vi "main_gui.vi"(8 "error in (no error)":errorcluster) -> (0 "error out":errorcluster)   [LabVIEW 2020]
uses:
  #typedefs/#typedef_cluster_GUI_QueueData.ctl
  #typedefs/#typedef_enum_GUI_States.ctl
  #typedefs/#typedef_enum_QueueActions.ctl
  #typedefs/#typedef_enum_EventActions.ctl
  <vilib>/Utility/miscctls.llb/LVBrowseOptionsTypeDef.ctl
  #typedefs/#typedef_cluster_GUI_Data.ctl
  <vilib>/vision/Image Controls.llb/IMAQ Image.ctl
  #typedefs/#typedef_cluster_CTRL_QueueData.ctl
  #typedefs/#typedef_enum_CTRL_States.ctl
panel:
  out "File Type":string
  in  "GenConsumerError":bool
  in  "GenProducerError":bool
  in  "Analyze Button":bool
  out "ImageName":string
  in  "Next Button":bool
  in  "Previous Button":bool
  out "ImagePreview":T1(plugin-control)
  in  "Add Button":bool
  in  "Select folder or image":path
  in  "Exit Button":bool
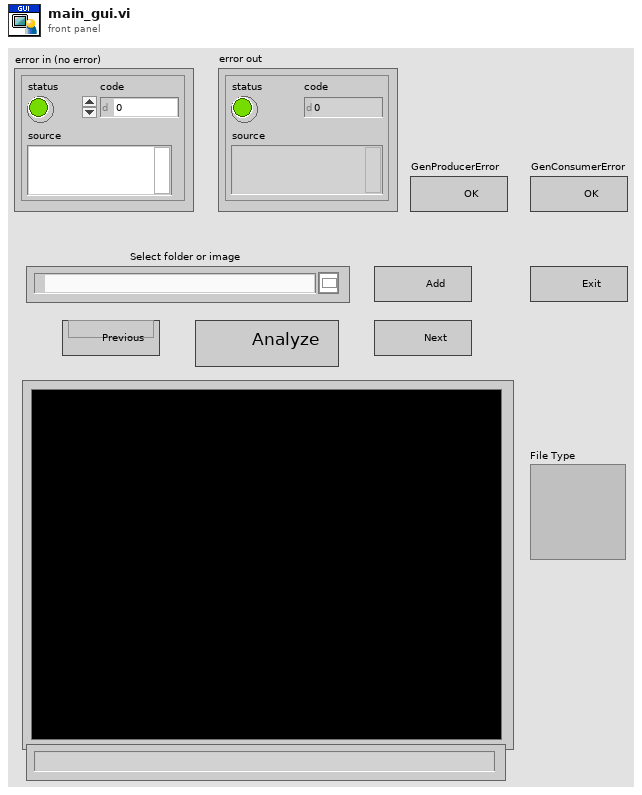
[diagram p1: front panel]
types:
  T1 = typedef "IMAQ Image.ctl" = refnum<image>
  T2 = typedef "#typedef_enum_EventActions.ctl" = enum16{"Obtain", "GetRef", "Generate", "Destroy"}
  T3 = typedef "#typedef_enum_QueueActions.ctl" = enum16{"Obtain", "GetRef", "Enqueue", "Release"}
  T4 = typedef "#typedef_cluster_GUI_QueueData.ctl" = cluster{"Cmd":T5, "Variant":variant}
  T5 = typedef "#typedef_enum_GUI_States.ctl" = enum16{"Init", "AddImages", "PreviousImage", "NextImage", "AnalyzeImage", "SaveImage", "GenFakeError", "ErrorHandling", "ExitRequest", "Exit"}
  T6 = enum32{"existing file", "new file", "new or existing file", "existing dir", "new dir", "new or existing dir", "existing file (use LLBs)", "new file (use LLBs)", "new or existing file (use LLBs)", "new or existing file or directory (use LLBs)", "existing dir (use LLBs)", "new dir (use LLBs)", "new or existing dir (use LLBs)", "existing file or dir", "new file or dir", "new or existing file or dir", "existing file or dir (use LLBs)", "new file or dir (use LLBs)"}
  T7 = typedef "LVBrowseOptionsTypeDef.ctl" = cluster{"Prompt":string, "Match Pattern":string, "Mode":enum32{"existing file", "new file", "new or existing file", "existing dir", "new dir", "new or existing dir", "existing file (use LLBs)", "new file (use LLBs)", "new or existing file (use LLBs)", "new or existing file or directory (use LLBs)", "existing dir (use LLBs)", "new dir (use LLBs)", "new or existing dir (use LLBs)", "existing file or dir", "new file or dir", "new or existing file or dir", "existing file or dir (use LLBs)", "new file or dir (use LLBs)"}, "Start Path":path, "Pattern Label":string, "Button Text":string}
  T8 = typedef "#typedef_enum_CTRL_States.ctl" = enum16{"Init", "AnalyzeImage", "SaveImage", "ErrorHandling", "ExitRequest", "Exit"}
  T9 = typedef "#typedef_cluster_CTRL_QueueData.ctl" = cluster{"Cmd":T8, "Variant":variant}
  T10 = typedef "#typedef_cluster_GUI_Data.ctl" = cluster{"Images":T1[], "PreviewIndex":i32, "AnalyzeIndex":i32, "Paths":path[]}
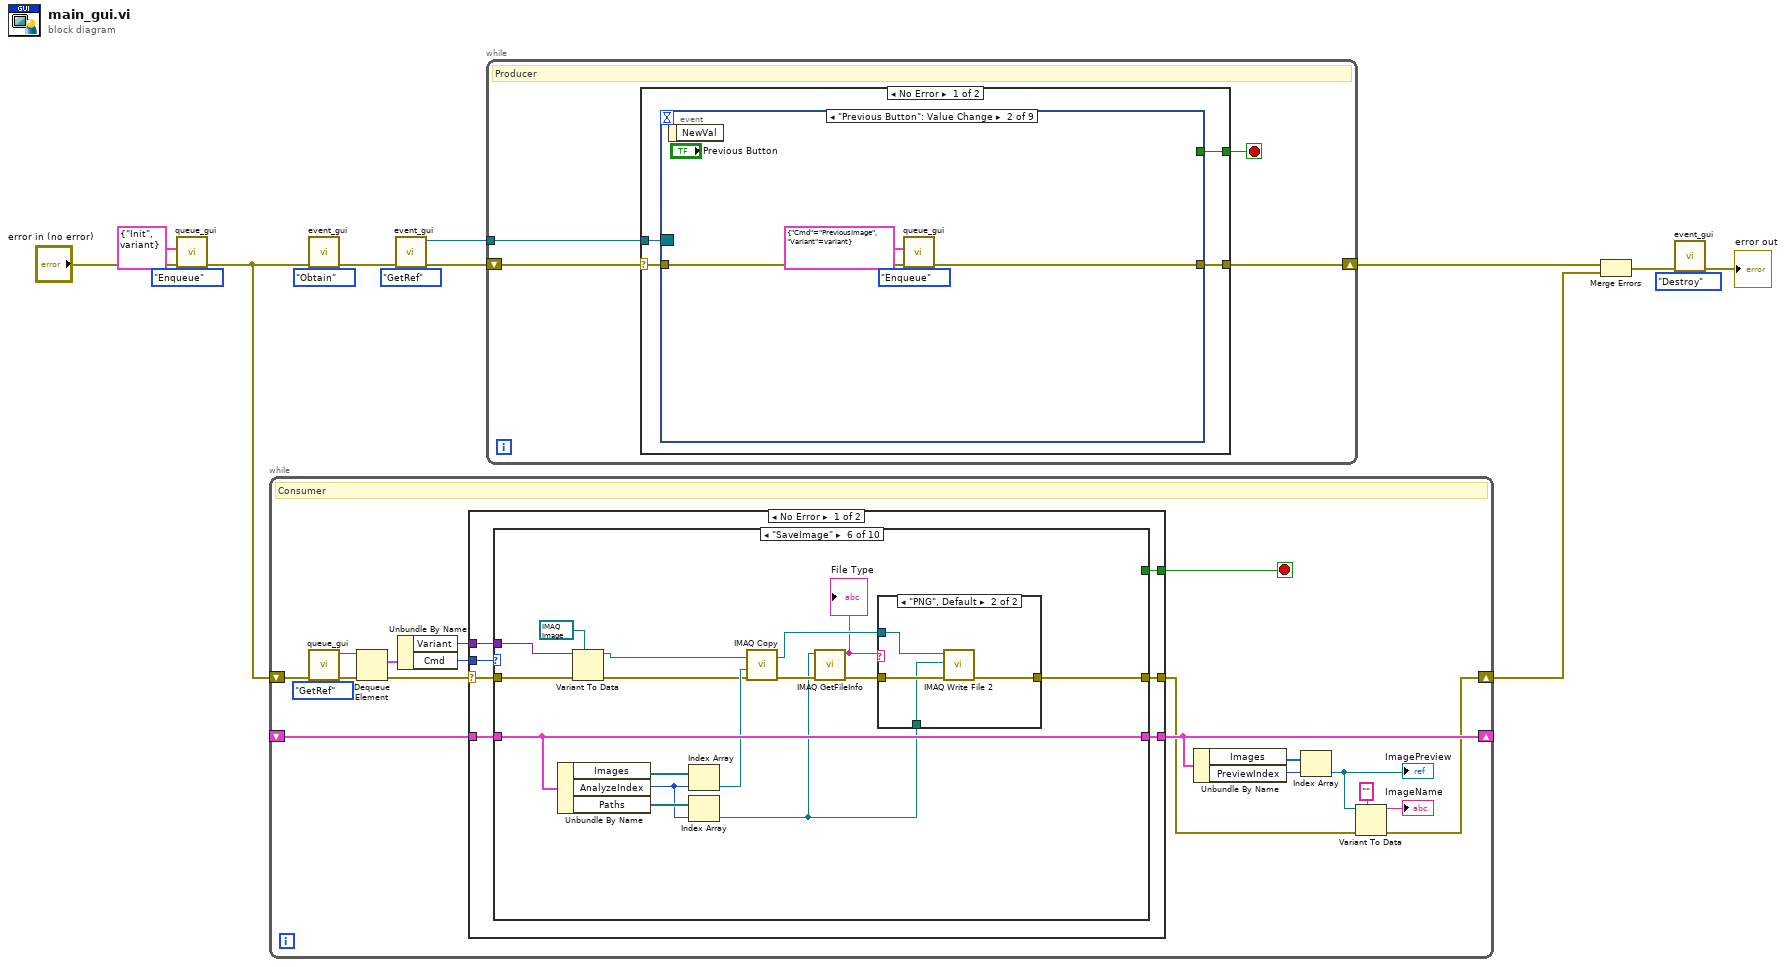
[diagram p0: block diagram]
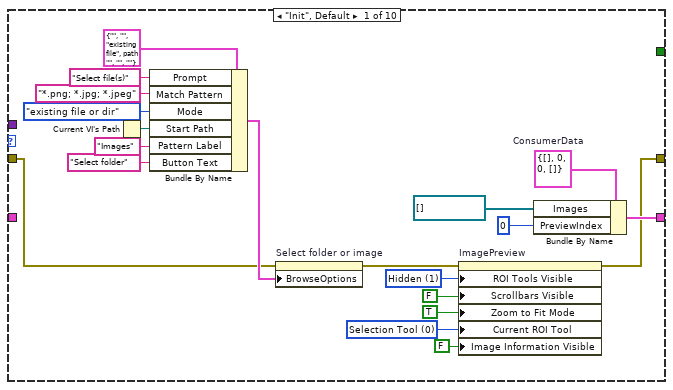
[diagram p2: hidden frame]
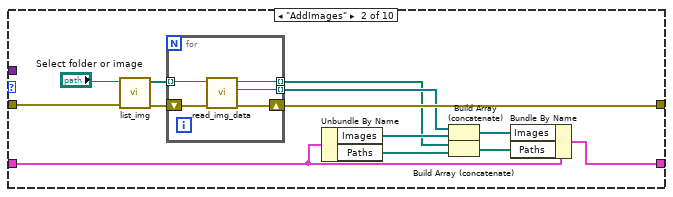
[diagram p3: hidden frame]
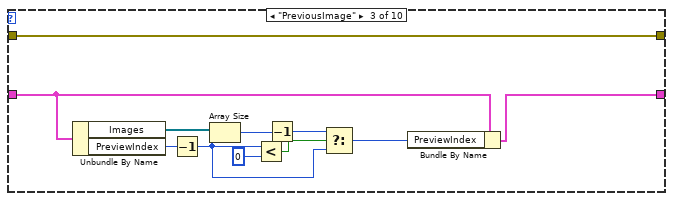
[diagram p4: hidden frame]
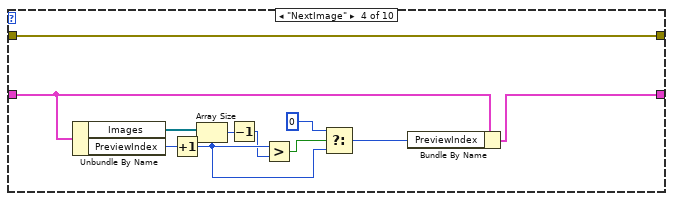
[diagram p5: hidden frame]
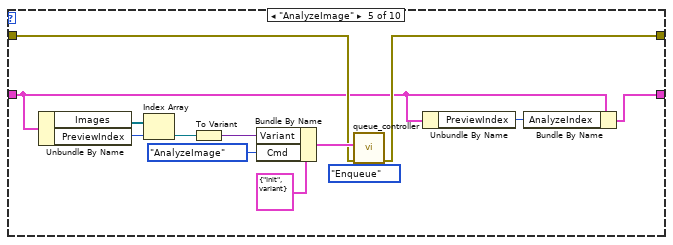
[diagram p6: hidden frame]
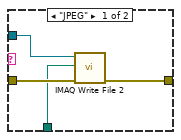
[diagram p7: hidden frame]
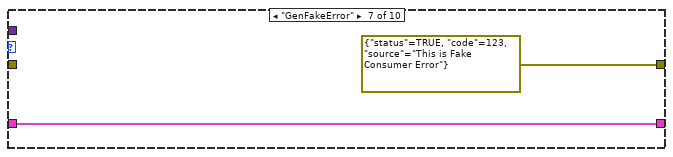
[diagram p8: hidden frame]
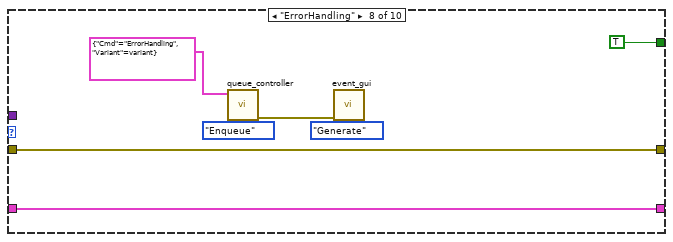
[diagram p9: hidden frame]
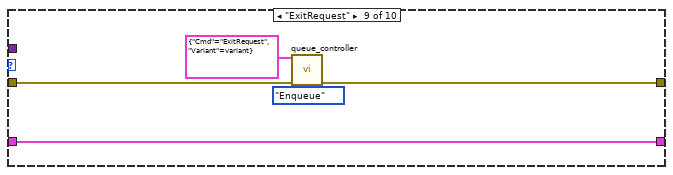
[diagram p10: hidden frame]
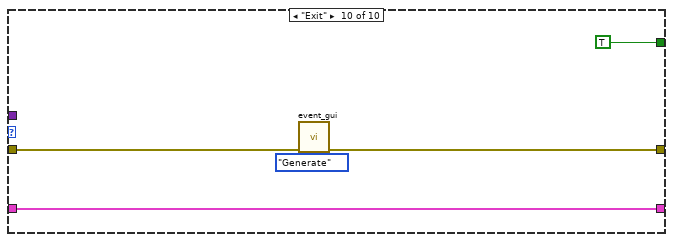
[diagram p11: hidden frame]
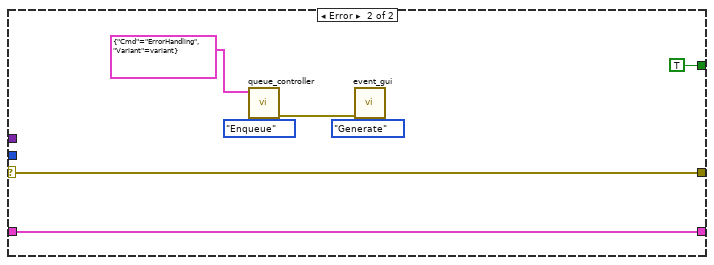
[diagram p12: hidden frame]
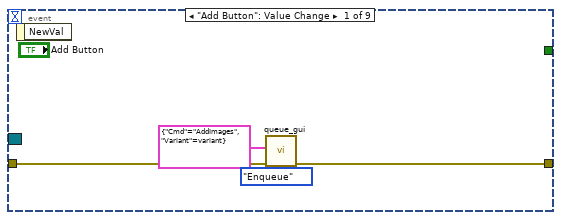
[diagram p13: hidden frame]
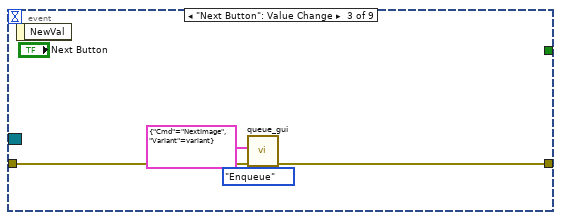
[diagram p14: hidden frame]
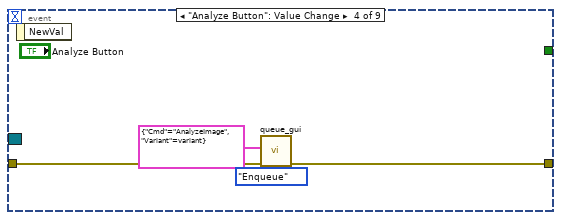
[diagram p15: hidden frame]
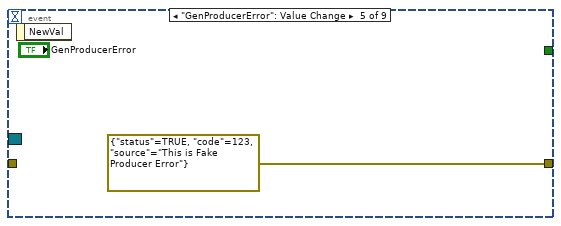
[diagram p16: hidden frame]
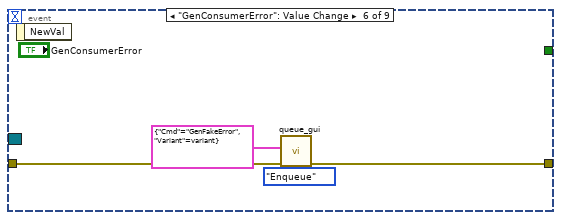
[diagram p17: hidden frame]
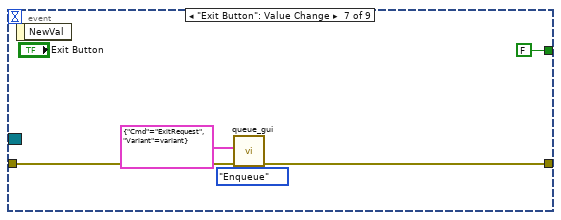
[diagram p18: hidden frame]
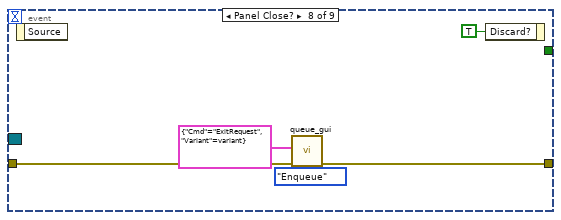
[diagram p19: hidden frame]
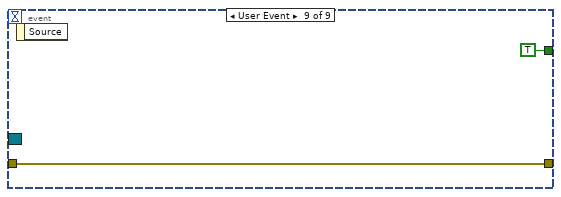
[diagram p20: hidden frame]
diagram:
  n1 = call "queue_gui.vi"("QueueActions"=#typedef_enum_QueueActions."Enqueue", "error in (no error)"="error in (no error)", "QueueDataIn"=T4 {"Cmd"=enum."Init", "Variant"=variant}) -> ("error out"=w4:errorcluster)  [unwired: 7 in, 1 out]
  n2 = while {
    shift-right: [w30] -> _
    shift-left: _ -> [w32]
    shift-right: [w23] -> w13
    shift-left: w4 -> [w22]
    stop <- w31 stop-if-true
    # "Consumer"
    n3 = call "queue_gui.vi"("QueueActions"=#typedef_enum_QueueActions."GetRef", "error in (no error)"=w22) -> ("error out"=w21:errorcluster, "queue out"=w19:refnum<queue>)  [unwired: 8 in]
    n4 = Dequeue Element(queue=w19, error in (no error)=w21) -> (element=w18:T4, error out=w16:errorcluster)  [unwired: 1 in, 2 out]
    n5 = Unbundle By Name(w18) -> ("Variant"=w15:variant, "Cmd"=w17:T5)
    n6 = case shown="No Error" w16 {
      selector: w16 -> [w34 w162]
      tunnel: w32 -> [w39 w161]
      tunnel: [w38 TRUE] -> w31
      tunnel: [w37 w161] -> w30
      tunnel: [w36 w162] -> w24
      tunnel: w17 -> [w35 _]
      tunnel: w15 -> [w33 _]
      frame No Error {
        n7 = case shown="\"SaveImage\"" w35 {
          tunnel: [w59 w69 w81 w94 w100 w124 w138 w145 w150 w155] -> w37
          tunnel: w39 -> [_ w70 w82 w95 w101 w124 w138 w145 w150 w155]
          tunnel: [w47 w68 w78 w89 w104 w120 errorcluster {"status"=TRUE, "code"=123, "source"="This is Fake Consumer Error"} ("error out") w140 w148 w152] -> w36
          tunnel: [_ _ _ _ _ _ _ TRUE _ TRUE] -> w38
          tunnel: w34 -> [w40 w63 w78 w89 w105 w128 _ w140 w149 w153]
          tunnel: w33 -> [_ _ _ _ _ w127 _ _ _ _]
          frame "Init", Default {
            w43 = u32 0 items=["Zoom Tool"=8, "Selection Tool"=0, "Pan Tool"=9, "Point Tool"=1, "Line Tool"=2, "Rectangle Tool"=3, "Rotated Rectangle Tool"=12, "Polyline Tool"=10, "Polygon Tool"=5, "Freehand Tool"=11, "Closed Freehand Tool"=6, "Ellipse Tool"=4, "Annulus Tool"=7] ("Current ROI Tool")
            w46 = u32 1 items=["Visible", "Hidden", "Hidden, Use WindTools Palette"] ("ROI Tools Visible")
            w50 = T10 {"Images"=[], "PreviewIndex"=0, "AnalyzeIndex"=0, "Paths"=[]}  # ConsumerData
            n8 = Current VI's Path() -> (path=w56:path)
            n9 = Bundle By Name(cluster=T7 {"Prompt"="", "Match Pattern"="", "Mode"=enum."existing file", "Start Path"=path "", "Pattern Label"="", "Button Text"=""} ("Browse Options"), "Prompt"="Select file(s)", "Match Pattern"="*.png; *.jpg; *.jpeg", "Mode"=T6."existing file or dir", "Start Path"=w56, "Pattern Label"="Images", "Button Text"="Select folder") -> (w52:T7)
            n10 = property on="Select folder or image" class="Path"(error in=w40, "BrowseOptions"=w52) -> (error out=w48:errorcluster)  [unwired: 1 in, 1 out]
            n11 = property on="ImagePreview" class="ImageControl"(error in=w48, "ROI Tools Visible"=w46, "Scrollbars Visible"=FALSE, "Zoom to Fit Mode"=TRUE, "Current ROI Tool"=w43, "Image Information Visible"=FALSE) -> (error out=w47:errorcluster)  [unwired: 1 in, 1 out]
            n12 = Bundle By Name(cluster=w50, "Images"=T1[] [], "PreviewIndex"=0 ("Progress")) -> (w59:T10)
          }
          frame "AddImages" {
            n13 = call "list_img.vi"("error in"=w63, "Input path"="Select folder or image") -> ("error out"=w71:errorcluster, "Output list of paths"=w72:path[])  [unwired: 8 in]
            n14 = for {
              tunnel: w72 -> [w75] mode=indexing
              shift-right: [w76] -> w68
              shift-left: w71 -> [w77]
              tunnel: [w74] -> w66 mode=indexing
              tunnel: [w73] -> w61 mode=indexing
              n15 = call "read_img_data.vi"("error in (no error)"=w77, "Input path"=w75) -> ("error out"=w76:errorcluster, "Image Out"=w74:T1, "Output path"=w73:path)  [unwired: 6 in]
            }
            n16 = Unbundle By Name(w70) -> ("Images"=w65:T1[], "Paths"=w60:path[])
            n17 = Build Array (concatenate)(w66, w65) -> (w64:T1[])
            n18 = Build Array (concatenate)(w61, w60) -> (w62:path[])
            n19 = Bundle By Name(cluster=w70, "Images"=w64, "Paths"=w62) -> (w69:T10)
          }
          frame "PreviousImage" {
            n20 = Unbundle By Name(w82) -> ("Images"=w88:T1[], "PreviewIndex"=w84:i32)
            n21 = Decrement(x=w84) -> (x-1=w80:i32)
            n22 = Array Size(array=w88) -> (size(s)=w85:i32)
            n23 = Less?(x=w80, y=0) -> (x < y?=w86:bool)
            n24 = Decrement(x=w85) -> (x-1=w79:i32)
            n25 = Select(t=w79, s=w86, f=w80) -> (s? t:f=w83:i32)
            n26 = Bundle By Name(cluster=w82, "PreviewIndex"=w83) -> (w81:T10)
          }
          frame "NextImage" {
            n27 = Unbundle By Name(w95) -> ("Images"=w99:T1[], "PreviewIndex"=w97:i32)
            n28 = Increment(x=w97) -> (x+1=w93:i32)
            n29 = Array Size(array=w99) -> (size(s)=w92:i32)
            n30 = Decrement(x=w92) -> (x-1=w90:i32)
            n31 = Greater?(x=w93, y=w90) -> (0:w98:bool)
            n32 = Select(t=0, s=w98, f=w93) -> (s? t:f=w96:i32)
            n33 = Bundle By Name(cluster=w95, "PreviewIndex"=w96) -> (w94:T10)
          }
          frame "AnalyzeImage" {
            n34 = Unbundle By Name(w101) -> ("Images"=w112:T1[], "PreviewIndex"=w111:i32)
            n35 = Index Array(array=w112, index=w111) -> (element=w110:T1)
            n36 = To Variant(anything=w110) -> (Variant=w107:variant)
            n37 = Bundle By Name(cluster=T9 {"Cmd"=enum."Init", "Variant"=variant} ("CTRL Data"), "Variant"=w107, "Cmd"=#typedef_enum_CTRL_States."AnalyzeImage") -> (w106:T9)
            n38 = call "queue_controller.vi"("QueueActions"=#typedef_enum_QueueActions."Enqueue", "error in (no error)"=w105, "QueueDataIn"=w106) -> ("error out"=w104:errorcluster)  [unwired: 7 in, 1 out]
            n39 = Unbundle By Name(w101) -> ("PreviewIndex"=w102:i32)
            n40 = Bundle By Name(cluster=w101, "AnalyzeIndex"=w102) -> (w100:T10)
          }
          frame "SaveImage" {
            n41 = Unbundle By Name(w124) -> ("Images"=w125:T1[], "AnalyzeIndex"=w118:i32, "Paths"=w119:path[])
            n42 = Variant To Data(error in=w128, type=T1 refnum ("element"), Variant=w127) -> (data=w121:T1, error out=w122:errorcluster)
            n43 = Index Array(array=w125, index=w118) -> (element=w123:T1)
            n44 = Index Array(array=w119, index=w118) -> (element=w115:path)
            n45 = call "IMAQ Copy"("error in (no error)"=w122, "Image Dst"=w123, "Image Src"=w121) -> ("error out"=w117:errorcluster, "Image Dst Out"=w114:T1)  [unwired: 3 in]
            n46 = call "IMAQ GetFileInfo"("error in (no error)"=w117, "File Path"=w115) -> ("error out"=w116:errorcluster, "File Type"=w113:string)  [unwired: 3 in, 5 out]
            "File Type" <- w113
            n47 = case shown="\"PNG\", Default" w113 {
              tunnel: [w132 w136] -> w120
              tunnel: w116 -> [w131 w135]
              tunnel: w115 -> [w130 w134]
              tunnel: w114 -> [w129 w133]
              frame "JPEG" {
                n48 = call-poly "IMAQ Write File 2"("error in (no error)"=w131, "File Path"=w130, "Image"=w129) -> ("error out"=w132:errorcluster)  [unwired: 7 in, 1 out]
              }
              frame "PNG", Default {
                n49 = call-poly "IMAQ Write File 2"("error in (no error)"=w135, "File Path"=w134, "Image"=w133) -> ("error out"=w136:errorcluster)  [unwired: 7 in, 1 out]
              }
            }
          }
          frame "GenFakeError" {
          }
          frame "ErrorHandling" {
            n50 = call "queue_controller.vi"("QueueActions"=#typedef_enum_QueueActions."Enqueue", "QueueDataIn"=T9 {"Cmd"=enum."ErrorHandling", "Variant"=variant}) -> ("error out"=w141:errorcluster)  [unwired: 8 in, 1 out]
            n51 = call "event_gui.vi"("EventAction"=#typedef_enum_EventActions."Generate", "error in (no error)"=w141) -> ()  [unwired: 8 in, 2 out]
          }
          frame "ExitRequest" {
            n52 = call "queue_controller.vi"("QueueActions"=#typedef_enum_QueueActions."Enqueue", "error in (no error)"=w149, "QueueDataIn"=T9 {"Cmd"=enum."ExitRequest", "Variant"=variant}) -> ("error out"=w148:errorcluster)  [unwired: 7 in, 1 out]
          }
          frame "Exit" {
            n53 = call "event_gui.vi"("EventAction"=#typedef_enum_EventActions."Generate", "error in (no error)"=w153) -> ("error out"=w152:errorcluster)  [unwired: 8 in, 1 out]
          }
        }
      }
      frame Error {
        n54 = call "queue_controller.vi"("QueueActions"=#typedef_enum_QueueActions."Enqueue", "QueueDataIn"=T9 {"Cmd"=enum."ErrorHandling", "Variant"=variant}) -> ("error out"=w157:errorcluster)  [unwired: 8 in, 1 out]
        n55 = call "event_gui.vi"("EventAction"=#typedef_enum_EventActions."Generate", "error in (no error)"=w157) -> ()  [unwired: 8 in, 2 out]
      }
    }
    n56 = Unbundle By Name(w30) -> ("Images"=w29:T1[], "PreviewIndex"=w28:i32)
    n57 = Index Array(array=w29, index=w28) -> (element=w25:T1)
    "ImagePreview" <- w25
    n58 = Variant To Data(error in=w24, type="", Variant=w25) -> (data=→"ImageName":string, error out=w23:errorcluster)
  }
  n59 = call "event_gui.vi"("EventAction"=#typedef_enum_EventActions."Obtain", "error in (no error)"=w4) -> ("error out"=w3:errorcluster)  [unwired: 8 in, 1 out]
  n60 = call "event_gui.vi"("EventAction"=#typedef_enum_EventActions."GetRef", "error in (no error)"=w3) -> ("error out"=w6:errorcluster, "Event Registration Refnum"=w7:refnum<event-registration>)  [unwired: 8 in]
  n61 = while {
    tunnel: w7 -> [w164]
    shift-right: [w165] -> w14
    shift-left: w6 -> [w163]
    stop <- w166 stop-if-true
    # "Producer"
    n62 = case shown="No Error" w163 {
      selector: w163 -> [w167 w207]
      tunnel: [w170 TRUE] -> w166
      tunnel: [w169 w207] -> w165
      tunnel: w164 -> [w168 _]
      frame No Error {
        n63 = event shown="[1] \"Previous Button\": Value Change" {
          selector: w168 -> [_ _ _ _ _ _ _ _ _]
          dyn-events: _ -> [_ _ _ _ _ _ _ _ _]
          timeout: _ -> [_ _ _ _ _ _ _ _ _]
          tunnel: [_ _ _ _ _ _ FALSE _ TRUE] -> w170
          tunnel: w167 -> [w174 w178 w182 w186 _ w189 w195 w198 w203]
          tunnel: [w173 w177 w181 w185 errorcluster {"status"=TRUE, "code"=123, "source"="This is Fake Producer Error"} ("error constant") w188 w194 w197 w203] -> w169
          event "Add Button": Value Change {
            n64 = event-data() -> ()  [unwired: 1 in, 1 out]
            n65 = call "queue_gui.vi"("QueueActions"=#typedef_enum_QueueActions."Enqueue", "error in (no error)"=w174, "QueueDataIn"=T4 {"Cmd"=enum."AddImages", "Variant"=variant} ("element")) -> ("error out"=w173:errorcluster)  [unwired: 7 in, 1 out]
          }
          event "Previous Button": Value Change {
            n66 = event-data() -> ()  [unwired: 1 in, 1 out]
            n67 = call "queue_gui.vi"("QueueActions"=#typedef_enum_QueueActions."Enqueue", "error in (no error)"=w178, "QueueDataIn"=T4 {"Cmd"=enum."PreviousImage", "Variant"=variant} ("element")) -> ("error out"=w177:errorcluster)  [unwired: 7 in, 1 out]
          }
          event "Next Button": Value Change {
            n68 = event-data() -> ()  [unwired: 1 in, 1 out]
            n69 = call "queue_gui.vi"("QueueActions"=#typedef_enum_QueueActions."Enqueue", "error in (no error)"=w182, "QueueDataIn"=T4 {"Cmd"=enum."NextImage", "Variant"=variant} ("element")) -> ("error out"=w181:errorcluster)  [unwired: 7 in, 1 out]
          }
          event "Analyze Button": Value Change {
            n70 = event-data() -> ()  [unwired: 1 in, 1 out]
            n71 = call "queue_gui.vi"("QueueActions"=#typedef_enum_QueueActions."Enqueue", "error in (no error)"=w186, "QueueDataIn"=T4 {"Cmd"=enum."AnalyzeImage", "Variant"=variant} ("element")) -> ("error out"=w185:errorcluster)  [unwired: 7 in, 1 out]
          }
          event "GenProducerError": Value Change {
            n72 = event-data() -> ()  [unwired: 1 in, 1 out]
          }
          event "GenConsumerError": Value Change {
            n73 = event-data() -> ()  [unwired: 1 in, 1 out]
            n74 = call "queue_gui.vi"("QueueActions"=#typedef_enum_QueueActions."Enqueue", "error in (no error)"=w189, "QueueDataIn"=T4 {"Cmd"=enum."GenFakeError", "Variant"=variant} ("element")) -> ("error out"=w188:errorcluster)  [unwired: 7 in, 1 out]
          }
          event "Exit Button": Value Change {
            n75 = event-data() -> ()  [unwired: 1 in, 1 out]
            n76 = call "queue_gui.vi"("QueueActions"=#typedef_enum_QueueActions."Enqueue", "error in (no error)"=w195, "QueueDataIn"=T4 {"Cmd"=enum."ExitRequest", "Variant"=variant} ("element")) -> ("error out"=w194:errorcluster)  [unwired: 7 in, 1 out]
          }
          event Panel Close? {
            n77 = event-data() -> ()  [unwired: 1 in, 1 out]
            n78 = call "queue_gui.vi"("QueueActions"=#typedef_enum_QueueActions."Enqueue", "error in (no error)"=w198, "QueueDataIn"=T4 {"Cmd"=enum."ExitRequest", "Variant"=variant} ("element")) -> ("error out"=w197:errorcluster)  [unwired: 7 in, 1 out]
            n79 = event-data("Discard?"=TRUE) -> ()  [unwired: 1 in, 1 out]
          }
          event User Event {
            n80 = event-data() -> ()  [unwired: 1 in, 1 out]
          }
        }
      }
      frame Error {
        n81 = call "queue_gui.vi"("QueueActions"=#typedef_enum_QueueActions."Enqueue", "QueueDataIn"=T4 {"Cmd"=enum."ErrorHandling", "Variant"=variant}) -> ()  [unwired: 8 in, 2 out]
      }
    }
  }
  n82 = Merge Errors(w14, w13) -> (w12:errorcluster)
  n83 = call "event_gui.vi"("EventAction"=#typedef_enum_EventActions."Destroy", "error in (no error)"=w12) -> ("error out"=→"error out":errorcluster)  [unwired: 8 in, 1 out]
